vi "lfw_people.vi"(8 "error in (no error)":errorcluster caption="entrée d'erreur (pas d'erreur)", 11 "fetch_lfw_people":T2={"funneled"=TRUE, "resize"=0.5, "min_faces_per_person"=0, "color"=FALSE, "slice_"={"Cluster"={"height"=70, "width"=195}, "Cluster 2"={"height"=78, "width"=172}}, "download_if_missing"=TRUE, "Returns"="Data"}) -> (0 "error out":errorcluster, 3 "Data":T1)   [LabVIEW 2020]
doc: "Face Recognition or Face Identification is: given the picture of the face of an unknown person, identify the name of the person by referring to a gallery of previously seen pictures of identified persons.\n\nData Set Characteristics : \n - Classes : 5749\n - Samples total : 13233\n - Dimensionality : 5828\n - Features : real, between 0 and 255\nParameters :\n\n- funneled : boolean, optional, default: True\nDownload and use the funneled variant of the dataset.\n\n- resize : float, optional, default 0.5\nRatio used to resize the each face picture.\n\n- min_faces_per_person : int, optional, default None\nThe extracted dataset will only retain pictures of people that have at least min_faces_per_person different pictures.\n\n- color : boolean, optional, default False\nKeep the 3 RGB channels instead of averaging them to a single gray level channel. If color is True the shape of the data has one more dimension than the shape with color = False.\n\n- slice_ : optional\nProvide a custom 2D slice (height, width) to extract the ‘interesting’ part of the jpeg files and avoid use statistical correlation from the background\n\n- download_if_missing : optional, True by default\nIf False, raise a IOError if the data is not locally available instead of trying to download the data from the source site.\n\n\nReturns : \n\n- data : numpy array of shape (13233, 62, 47)\nEach row is a face image corresponding to one of the 5749 people in the dataset. Changing the slice_ or resize parameters will change the shape of the output.\n\n- target : numpy array of shape (13233,)\nLabels associated to each face image. Those labels range from 0-5748 and correspond to the person IDs."
uses:
  lfw_people.lvclass
panel:
  out "lfw_people.lvclass":refnum<class "lfw_people.lvclass">
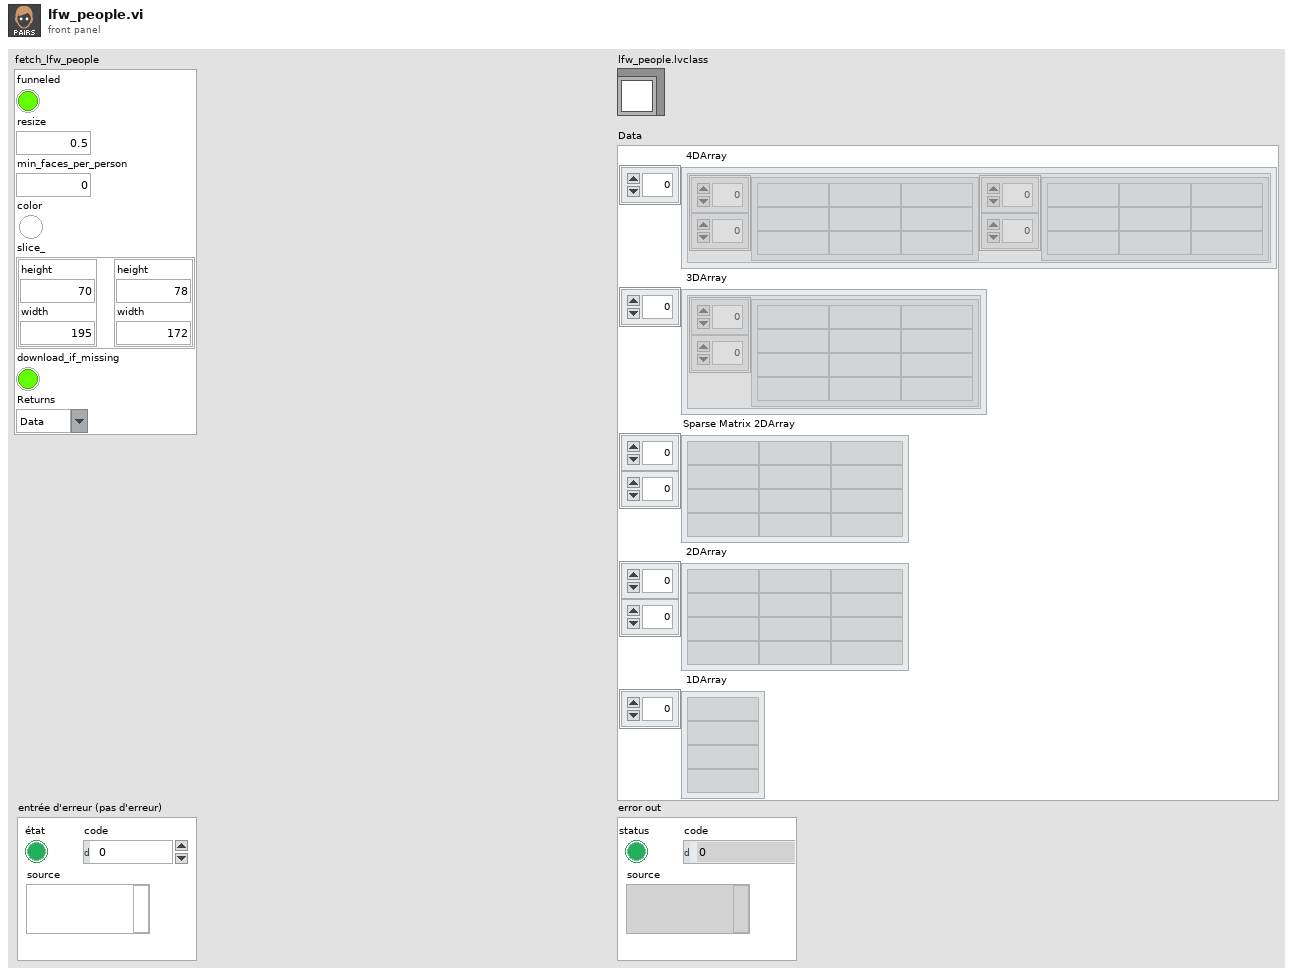
[diagram p1: front panel]
types:
  T1 = cluster{" 4DArray":cluster{"1":string[][], "2":string[][]}[], " 3DArray":cluster{"Tableau":string[][]}[], "Sparse Matrix 2DArray":string[][], " 2DArray":string[][], " 1DArray":string[]}
  T2 = cluster{"funneled":bool, "resize":dbl, "min_faces_per_person":i32, "color":bool, "slice_":cluster{"Cluster":cluster{"height":u32, "width":u32}, "Cluster 2":cluster{"height":u32, "width":u32}}, "download_if_missing":bool, "Returns":string}
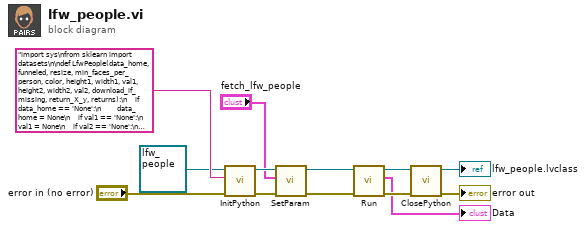
[diagram p0: block diagram]
diagram:
  n1 = call-dynamic "InitPython.vi"("error in (no error)"="error in (no error)", "Python Instruction"="import sys\nfrom sklearn import datasets\n\ndef LfwPeople(data_home, funneled, resize, min_faces_per_person, color, height1, width1, val1, height2, width2, val2, download_if_missing, return_X_y, returns):\n    if data_home == 'None':\n        data_home = None\n    if val1 == 'None':\n        val1 = None\n    if val2 == 'None':\n        val2 = None\n    try:\n        LfwPeople = datasets.fetch_lfw_people(data_home, funneled, resize, min_faces_per_person, color, (slice(height1, width1, val1), slice(height2, width2, val2)), download_if_missing, return_X_y)\n        if returns == 'Data': \n            data = LfwPeople['images'].tolist()\n            return str(data)\n        else :\n            data = LfwPeople['target'].tolist()\n            return str(data)\n    except:\n        erreur = sys.exc_info()\n        typerr = u\"%s\" % (erreur[0])\n        typerr = typerr[typerr.find(\"'\")+1:typerr.rfind(\"'\")]\n        msgerr = u\"%s\" % (erreur[1])\n        message = str('/!\\\\ {0} : {1}'. format(typerr,msgerr))\n        return message", "Scikit-learn en entrée"=refnum<class "lfw_people.lvclass"> refnum ("lfw_people.lvclass")) -> ("error out"=w9:errorcluster, "Scikit-learn en sortie"=w10:refnum<class "lfw_people.lvclass">)  [unwired: 7 in]
  n2 = call-dynamic "SetParam.vi"("error in"=w9, "fetch_lfw_people"="fetch_lfw_people", "lfw_people.lvclass"=w10) -> ("error out"=w6:errorcluster, "lfw_people.lvclass"=w7:refnum<class "lfw_people.lvclass">)  [unwired: 7 in]
  n3 = call-dynamic "Run.vi"("error in"=w6, "lfw_people.lvclass"=w7) -> ("error out"=w4:errorcluster, "Data"=→"Data":T1, "lfw_people.lvclass"=w5:refnum<class "lfw_people.lvclass">)  [unwired: 7 in]
  n4 = call-dynamic "ClosePython.vi"("error in (no error)"=w4, "Scikit-learn en entrée"=w5) -> ("error out"=→"error out":errorcluster, "Scikit-learn en sortie"=→"lfw_people.lvclass":refnum<class "lfw_people.lvclass">)  [unwired: 8 in]
